vi "Replace Template Clusters.vi"(6 "Traverse Target":T1=enum."BD", 8 "error in (no error)":errorcluster, 9 "Control Name":string="Compiled.Settings", 10 "Path to Cluster to Replace":path, 11 "Path to VI":path) -> (0 "error out":errorcluster)   [LabVIEW 2015]
doc: "This VI allows you to replace template clusters, on either the FP or BD, with a new cluster control by name."
uses:
  <vilib>/Utility/traverseref.llb/TRef TravTarget.ctl
  <vilib>/Utility/traverseref.llb/VI Scripting - Traverse.lvlib
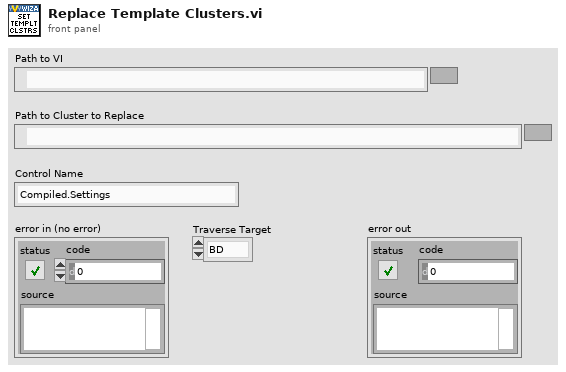
[diagram p1: front panel]
types:
  T1 = typedef "TRef TravTarget.ctl" = enum16{"FP", "BD", "Other"}
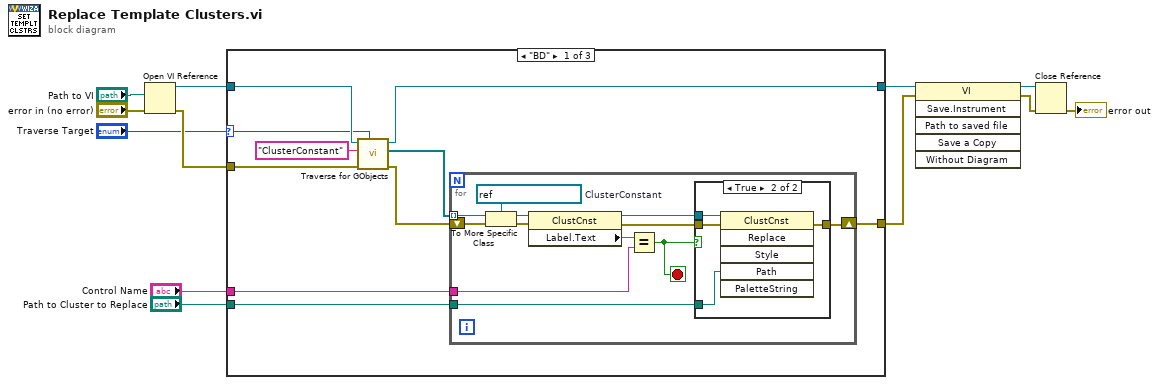
[diagram p0: block diagram]
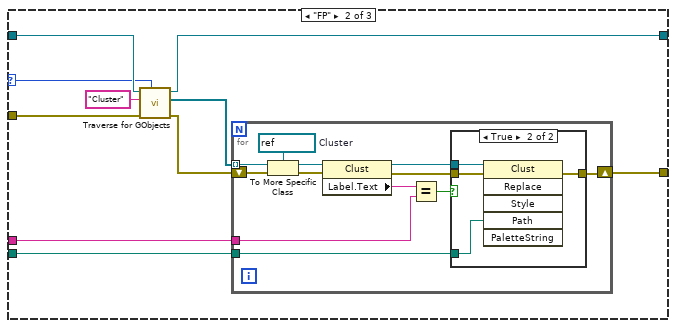
[diagram p3: hidden frame]
diagram:
  n1 = Open VI Reference(vi path="Path to VI", error in (no error)="error in (no error)") -> (vi reference=w4:refnum<vi>, error out=w5:errorcluster)  [unwired: 4 in]
  n2 = case shown="\"BD\"" "Traverse Target" {
    selector: "Traverse Target" -> [w13 w40 _]
    tunnel: "Path to Cluster to Replace" -> [w22 w49 _]
    tunnel: [w21 w48 w67] -> w10
    tunnel: [w20 w47 w68] -> w6
    tunnel: w5 -> [w19 w46 w67]
    tunnel: w4 -> [w18 w45 w68]
    tunnel: "Control Name" -> [w17 w44 _]
    frame "BD" {
      n3 = call <vilib>:"Traverse for GObjects.vi"("Traverse Target"=w13, "error in (no error)"=w19, "Class Name"="ClusterConstant", "VI Refnum"=w18) -> ("error out"=w15:errorcluster, "References"=w14:refnum<vi>[], "dup VI Refnum"=w20:refnum<vi>)  [unwired: 4 in, 1 out]
      n4 = for {
        tunnel: w14 -> [w34] mode=indexing
        shift-right: [w24] -> w21
        shift-left: w15 -> [w32]
        tunnel: w17 -> [w28]
        tunnel: w22 -> [w25]
        stop <- w23 stop-if-true
        w33 = refnum<vi> refnum  # ClusterConstant
        n5 = To More Specific Class(target class=w33, reference=w34, error in=w32) -> (specific class reference=w31:refnum<vi>, error out=w30:errorcluster)
        n6 = property class="ClustCnst"(reference=w31, error in=w30) -> (reference out=w27:refnum<vi>, error out=w26:errorcluster, "Label.Text"=w29:string)
        n7 = Equal?(x=w29, y=w28) -> (x = y?=w23:bool)
        n8 = case shown="True" w23 {
          tunnel: w27 -> [_ w39]
          tunnel: w26 -> [w35 w38]
          tunnel: w25 -> [_ w37]
          tunnel: [w35 w36] -> w24
          frame False {
          }
          frame True {
            n9 = invoke class="ClustCnst" method="Replace"(reference=w39, error in=w38, "Path"=w37) -> (error out=w36:errorcluster)  [unwired: 3 in, 5 out]
          }
        }
      }
    }
    frame "FP" {
      n10 = call <vilib>:"Traverse for GObjects.vi"("Traverse Target"=w40, "error in (no error)"=w46, "Class Name"="Cluster", "VI Refnum"=w45) -> ("error out"=w42:errorcluster, "References"=w41:refnum<vi>[], "dup VI Refnum"=w47:refnum<vi>)  [unwired: 4 in, 1 out]
      n11 = for {
        tunnel: w41 -> [w61] mode=indexing
        shift-right: [w50] -> w48
        shift-left: w42 -> [w59]
        tunnel: w44 -> [w55]
        tunnel: w49 -> [w51]
        w60 = refnum<vi> refnum  # Cluster
        n12 = To More Specific Class(target class=w60, reference=w61, error in=w59) -> (specific class reference=w58:refnum<vi>, error out=w57:errorcluster)
        n13 = property class="Clust"(reference=w58, error in=w57) -> (reference out=w53:refnum<vi>, error out=w52:errorcluster, "Label.Text"=w56:string)
        n14 = Equal?(x=w56, y=w55) -> (x = y?=w54:bool)
        n15 = case shown="True" w54 {
          tunnel: w53 -> [_ w66]
          tunnel: w52 -> [w62 w65]
          tunnel: w51 -> [_ w64]
          tunnel: [w62 w63] -> w50
          frame False {
          }
          frame True {
            n16 = invoke class="Clust" method="Replace"(reference=w66, error in=w65, "Path"=w64) -> (error out=w63:errorcluster)  [unwired: 3 in, 5 out]
          }
        }
      }
    }
    frame "Other" {
    }
  }
  n17 = invoke class="VI" method="Save.Instrument"(reference=w6, error in=w10) -> (reference out=w7:refnum<vi>, error out=w8:errorcluster)  [unwired: 4 in, 4 out]
  n18 = Close Reference(reference=w7, error in (no error)=w8) -> (error out=→"error out":errorcluster)
